vi "Single Digit Tables.vi"() -> (3 "Map":map{i32, T1[]}(c390))   [LabVIEW 2024]
uses:
  Cluster_Blink result.ctl
panel:
  out "jump":i32
  out "number":i32
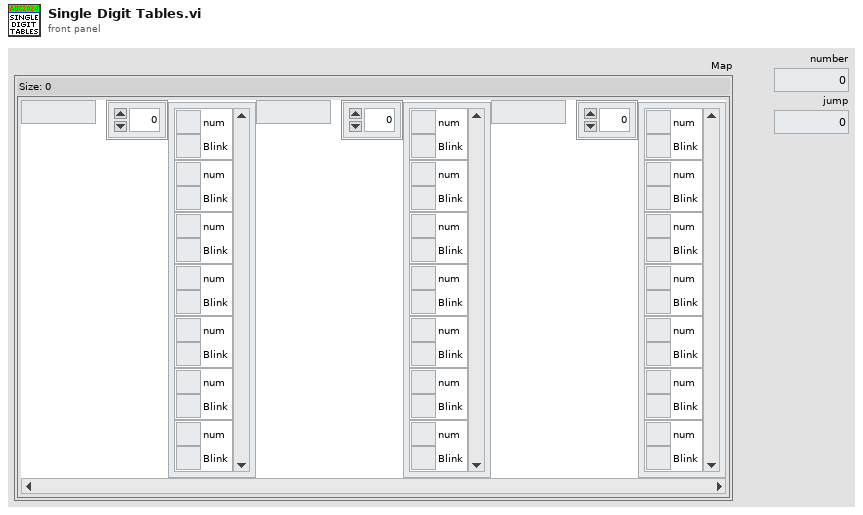
[diagram p1: front panel]
types:
  T1 = typedef "Cluster_Blink result.ctl" = cluster{"num":u64, "Blink":u64}
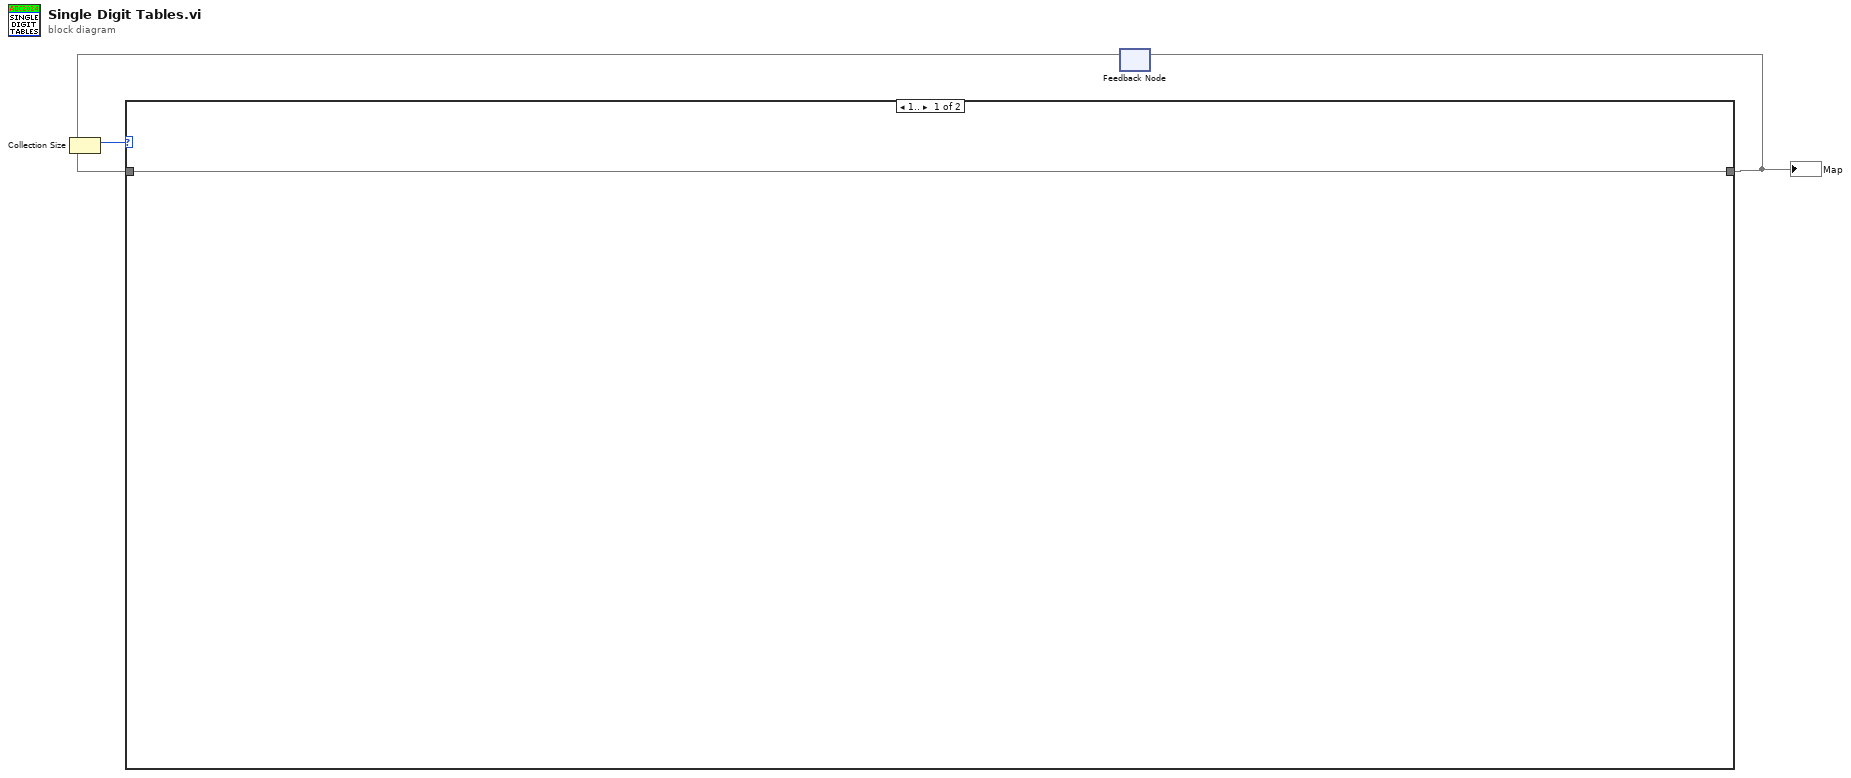
[diagram p0: block diagram]
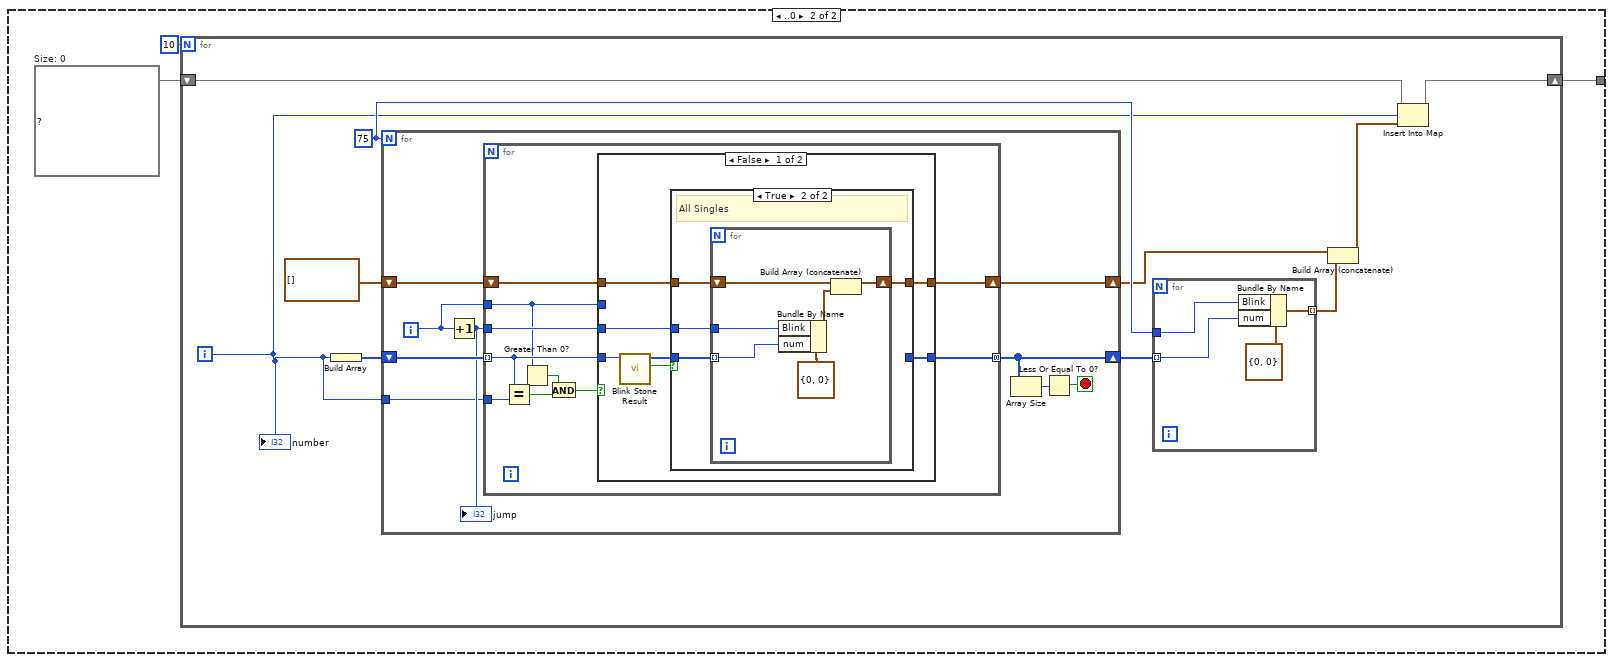
[diagram p2: hidden frame]
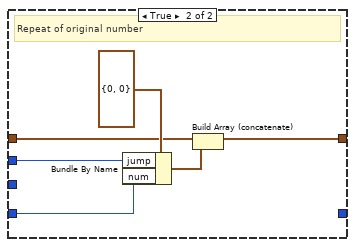
[diagram p4: hidden frame]
diagram:
  n1 = feedback #1() -> (w1:map{i32, T1[]})  [unwired: 1 in]
  n2 = Collection Size(1:w1) -> (0:w2:i32)
  n3 = case shown="1.." w2 {
    tunnel: [w4 w5] -> w3
    tunnel: w1 -> [w4 _]
    frame 1.. {
    }
    frame ..0 {
      w6 = map{i32, T1[]} {}  # Size: 0
      n4 = for {
        N: 10 -> [_]
        shift-right: [w15] -> w5
        shift-left: w6 -> [w16]
        i -> [w8]
        w12 = 75
        n5 = Build Array(w8) -> (w17:i32[])
        n6 = for {
          N: w12 -> [_]
          shift-right: [w26] -> w13
          shift-left: w17 -> [w30]
          shift-right: [w27] -> w11
          shift-left: T1[] [] -> [w28]
          tunnel: w8 -> [w23]
          i -> [w24]
          stop <- w22 stop-if-true
          n7 = Increment(x=w24) -> (x+1=w29:i32)
          "jump" <- w29
          n8 = for {
            tunnel: w30 -> [w36] mode=indexing
            tunnel: w29 -> [w38]
            shift-right: [w37] -> w27
            shift-left: w28 -> [w40]
            tunnel: [w39] -> w26 mode=concatenating
            tunnel: w24 -> [w31]
            tunnel: w23 -> [w35]
            n9 = Equal?(x=w36, y=w35) -> (x = y?=w34:bool)
            n10 = Greater Than 0?(x=w31) -> (x > 0?=w32:bool)
            n11 = And(x=w32, y=w34) -> (x .and. y?=w33:bool)
            n12 = case shown="False" w33 {
              tunnel: w40 -> [w45 w62]
              tunnel: [w44 _] -> w39
              tunnel: w38 -> [w43 _]
              tunnel: [w42 w61] -> w37
              tunnel: w36 -> [w41 w64]
              tunnel: w31 -> [_ w63]
              frame False {
                n13 = call "Blink Stone Result.vi"("String"=w41) -> ("Single Digits"=w47:bool, "Result Array"=w46:u64[])  [unwired: 9 in]
                n14 = case shown="True" w47 {
                  tunnel: w46 -> [w49 w53]
                  tunnel: w45 -> [w48 w51]
                  tunnel: [w49 _] -> w44
                  tunnel: w43 -> [_ w52]
                  tunnel: [w48 w50] -> w42
                  frame False {
                    # "Not Singles"
                  }
                  frame True {
                    # "All Singles"
                    n15 = for {
                      tunnel: w53 -> [w58] mode=indexing
                      tunnel: w52 -> [w57]
                      shift-right: [w54] -> w50
                      shift-left: w51 -> [w56]
                      n16 = Bundle By Name(cluster=T1 {"num"=0, "Blink"=0} ("Cluster"), "Blink"=w57, "num"=w58) -> (w55:T1)
                      n17 = Build Array (concatenate)(w56, w55) -> (w54:T1[])
                    }
                  }
                }
              }
              frame True {
                # "Repeat of original number"
                n18 = Bundle By Name(cluster=cluster{"num":i32, "jump":i32} {"num"=0, "jump"=0} ("Cluster"), "jump"=w63, "num"=w64) -> (w60:cluster{"num":i32, "jump":i32})
                n19 = Build Array (concatenate)(w62, w60) -> (w61:T1[])
              }
            }
          }
          n20 = Array Size(array=w26) -> (size(s)=w25:i32)
          n21 = Less Or Equal To 0?(x=w25) -> (x <= 0?=w22:bool)
        }
        n22 = for {
          tunnel: w13 -> [w20] mode=indexing
          tunnel: w12 -> [w19]
          tunnel: [w18] -> w10 mode=indexing
          n23 = Bundle By Name(cluster=T1 {"num"=0, "Blink"=0} ("Cluster"), "Blink"=w19, "num"=w20) -> (w18:T1)
        }
        n24 = Build Array (concatenate)(w11, w10) -> (w9:T1[])
        n25 = Insert Into Map(map in=w16, key=w8, value=w9) -> (map out=w15:map{i32, T1[]})  [unwired: 2 out]
        "number" <- w8
      }
    }
  }
  "Map" <- w3
  n26 = feedback-in #1(w3) -> ()
